vi "SSC Digital Burst Pattern [Pass Fail].vi"(0 "Digital SSC in":T1[](array[typedef]), 1 "Start Label":string, 2 "select digital function?":bool=TRUE caption="select digital function? (T)", 7 "timeout (s)":dbl=10.0, 11 "error in":errorcluster) -> (4 "Digital SSC out":T1[](array[typedef]), 6 "Per-Instrument Pass":bool[][](array[boolean]), 15 "error out":errorcluster)   [LabVIEW 2020]
doc: "Uses the start label you specify to burst the pattern on the pin(s) and pin group(s) you specify, waits for the burst to complete, and returns comparison results for each site."
uses:
  SSC Digital.ctl
  <instrlib>/niDigital/niDigital.llb/niDigital Burst Pattern (Pass Fail).vi
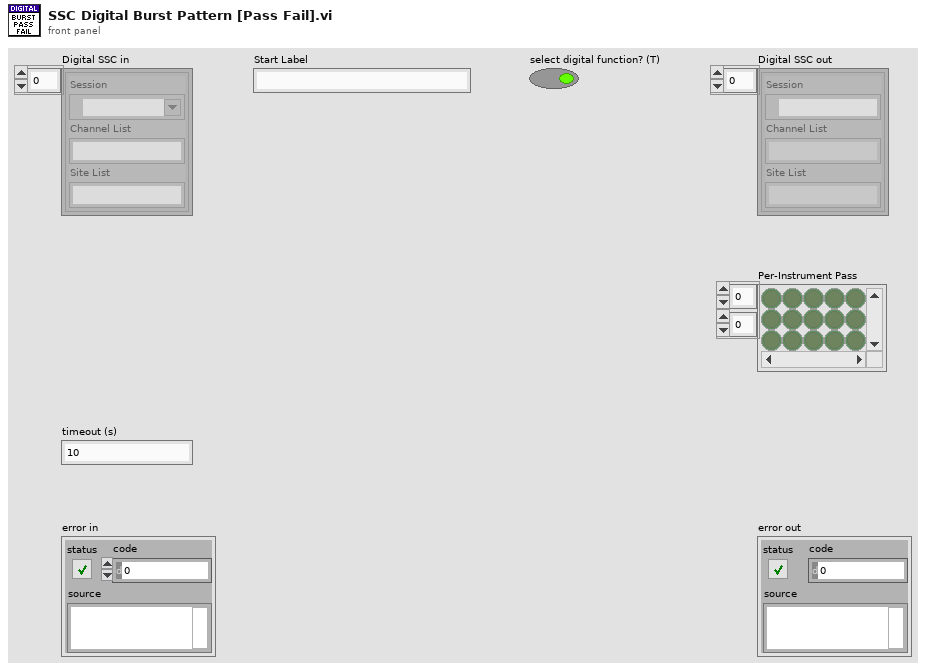
[diagram p1: front panel]
types:
  T1 = typedef "SSC Digital.ctl" = cluster{"Session":refnum<k15>, "Channel List":string, "Site List":string}
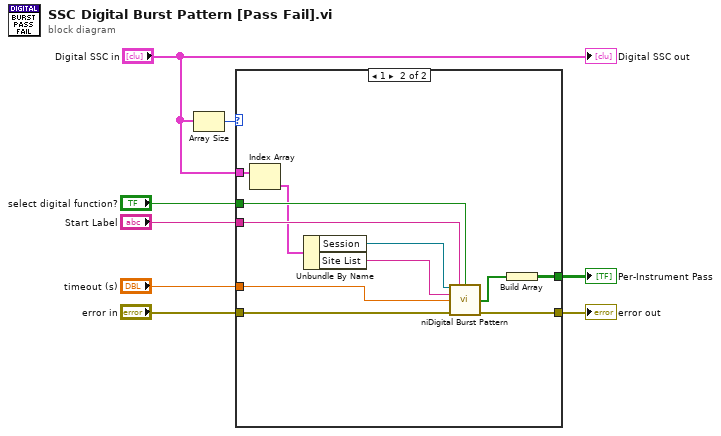
[diagram p0: block diagram]
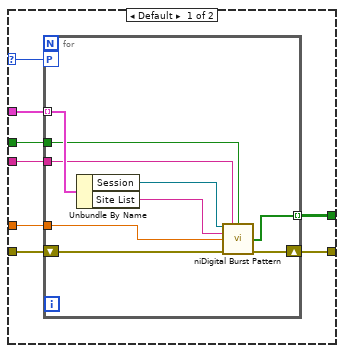
[diagram p2: hidden frame]
diagram:
  n1 = Array Size(array="Digital SSC in") -> (size(s)=w2:i32)
  n2 = case shown="1" w2 {
    selector: w2 -> [w10 _]
    tunnel: "Start Label" -> [w16 w36]
    tunnel: "select digital function?" -> [w15 w35]
    tunnel: "timeout (s)" -> [w14 w34]
    tunnel: "error in" -> [w13 w33]
    tunnel: [w12 w32] -> w4
    tunnel: [w11 w26] -> w3
    tunnel: "Digital SSC in" -> [w9 w30]
    frame Default {
      n3 = for {
        tunnel: w9 -> [w25] mode=indexing
        tunnel: w16 -> [w24]
        tunnel: w15 -> [w23]
        workers-P: w10 -> [_]
        tunnel: w14 -> [w20]
        shift-right: [w21] -> w12
        shift-left: w13 -> [w22]
        tunnel: [w17] -> w11 mode=indexing
        n4 = Unbundle By Name(w25) -> ("Session"=w19:refnum<k15>, "Site List"=w18:string)
        n5 = call-poly <instrlib>:"niDigital Burst Pattern.vi"("instrument handle"=w19, "start label"=w24, "select digital function? (T)"=w23, "site list"=w18, "timeout (s)"=w20, "error in"=w22) -> ("pass"=w17:bool[], "error out"=w21:errorcluster)  [unwired: 7 in, 1 out]
      }
    }
    frame 1 {
      n6 = Index Array(array=w30) -> (element=w27:T1)  [unwired: 1 in]
      n7 = Unbundle By Name(w27) -> ("Session"=w29:refnum<k15>, "Site List"=w28:string)
      n8 = call-poly <instrlib>:"niDigital Burst Pattern.vi"("instrument handle"=w29, "start label"=w36, "select digital function? (T)"=w35, "site list"=w28, "timeout (s)"=w34, "error in"=w33) -> ("pass"=w31:bool[], "error out"=w32:errorcluster)  [unwired: 7 in, 1 out]
      n9 = Build Array(w31) -> (w26:bool[][])
    }
  }
  "error out" <- w4
  "Per-Instrument Pass" <- w3
  "Digital SSC out" <- "Digital SSC in"
